vi "GET Full Save Path.vi"() -> (0 "Full Save Path":path)   [LabVIEW 2013]
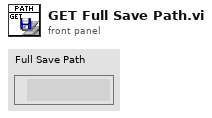
[diagram p1: front panel]
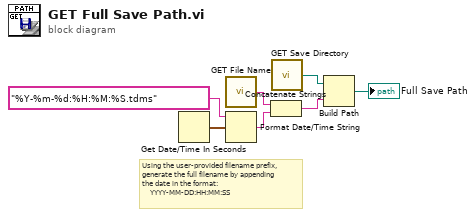
[diagram p0: block diagram]
diagram:
  # "Using the user-provided filename prefix,\ngenerate the full filename by appending \nthe date in the format:\n    YYYY-MM-DD:HH:MM:SS"
  n1 = Get Date/Time In Seconds() -> (seconds since 1Jan1904=w7:timestamp)
  n2 = call "GET File Name.vi"() -> ("File Name"=w4:string)
  n3 = Format Date/Time String(time format string (%c)="%Y-%m-%d:%H:%M:%S.tdms", seconds (now)=w7) -> (date/time string=w5:string)  [unwired: 1 in]
  n4 = Concatenate Strings(w4, w5) -> (w2:string)
  n5 = call "GET Save Directory.vi"() -> ("Save Directory"=w3:path)
  n6 = Build Path(base path=w3, name or relative path=w2) -> (appended path=→"Full Save Path":path)
